vi "RefToBool.vi"(6 "BoolRef":refnum<vi>) -> (1 "Boolen":bool, 2 "BoolRefOut":refnum<vi>)   [LabVIEW 2013]
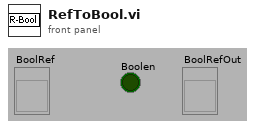
[diagram p1: front panel]
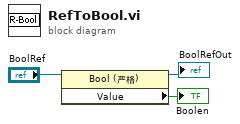
[diagram p0: block diagram]
diagram:
  n1 = property class="Bool (严格)"(reference="BoolRef") -> (reference out=→"BoolRefOut":refnum<vi>, "Value"=→"Boolen":bool)  [unwired: 1 in, 1 out]
